vi "systemErrorClusterReplacementCore.vi"(8 "error in (no error)":errorcluster, 11 "Folder Path":path) -> (0 "error out":errorcluster)   [LabVIEW 2017, in "vi_tools.lvlib"]
doc: "From the front panel or block diagram window of a VI or a VI is selected on the File Dialog, select <b>Tools»System Error Cluster Replacement</b> to replace all Error clusters (in and out) on the VI front panel with System Error cluster.\n\nFrom the a project or lvlib explorer window or a folder is selected on the File Dialog, select <b>Tools»System Error Cluster Replacement</b> to replace all Error clusters (in and out) on all VI front panels with System Error cluster within the project or lvlib or user selected folder on disk."
uses:
  <vilib>/Utility/traverseref.llb/TRef TravTarget.ctl
  vi_tools.lvlib
panel:
  out "progress":string
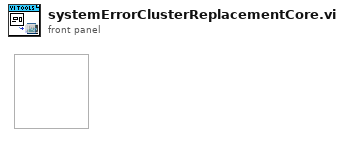
[diagram p1: front panel]
types:
  T1 = enum32{"Invalid", "Standard", "Closed", "Hidden", "Minimized", "Maximized"}
  T2 = typedef "TRef TravTarget.ctl" = enum16{"FP", "BD", "Other"}
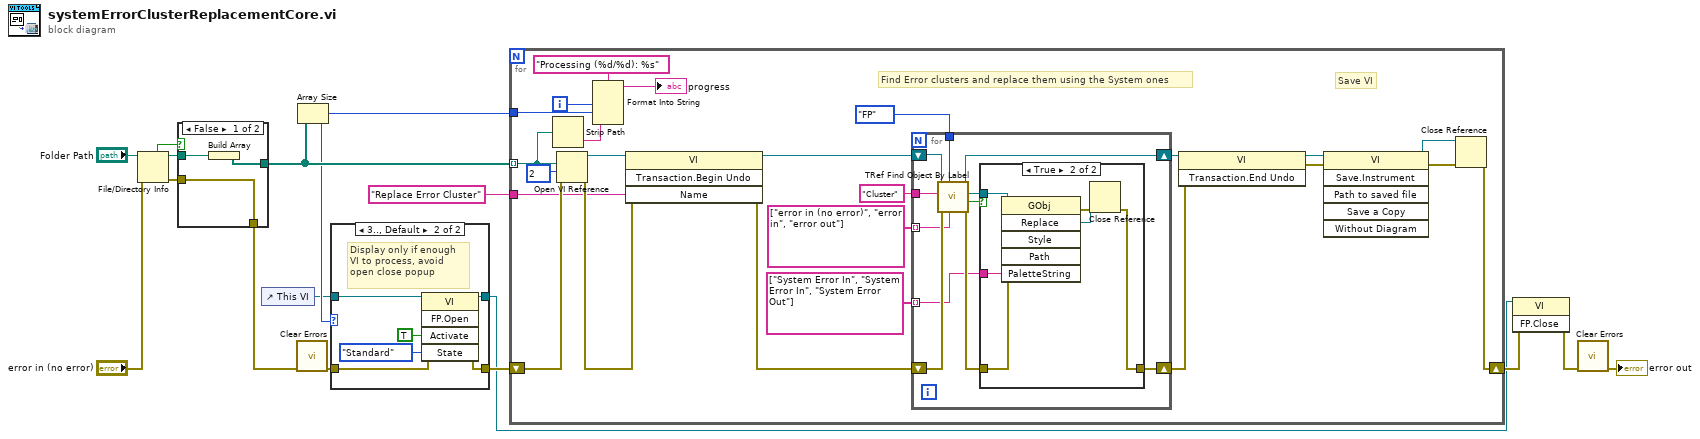
[diagram p0: block diagram]
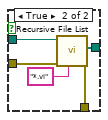
[diagram p2: hidden frame]
diagram:
  n1 = File/Directory Info(path="Folder Path", error in="error in (no error)") -> (path out=w10:path, directory=w8:bool, error out=w9:errorcluster)  [unwired: 4 out]
  n2 = case shown="False" w8 {
    tunnel: [w17 w23] -> w16
    tunnel: [w18 w22] -> w15
    tunnel: w10 -> [w19 w21]
    tunnel: w9 -> [w18 w20]
    frame False {
      n3 = Build Array(w19) -> (w17:path[])
    }
    frame True {
      n4 = call <vilib>:"Recursive File List.vi"("pattern"="*.vi", "error in (no error)"=w20, "Folder Path"=w21) -> ("error out"=w22:errorcluster, "All Files in Dir"=w23:path[])  [unwired: 4 in, 3 out]
    }
  }
  n5 = control-ref of="This VI"() -> (w2:refnum<vi>)
  n6 = call <vilib>:"Clear Errors.vi"("error in (no error)"=w15) -> ("error out"=w3:errorcluster)  [unwired: 5 in, 1 out]
  n7 = Array Size(array=w16) -> (size(s)=w4:i32)
  n8 = case shown="3.., Default" w4 {
    tunnel: w3 -> [w26 w30]
    tunnel: [w26 w29] -> w14
    tunnel: w2 -> [w25 w28]
    tunnel: [w25 w27] -> w5
    frame 0..2 {
    }
    frame 3.., Default {
      # "Display only if enough\nVI to process, avoid \nopen close popup"
      n9 = invoke class="VI" method="FP.Open"(reference=w28, error in=w30, "Activate"=TRUE ("Activate?"), "State"=T1."Standard") -> (reference out=w27:refnum<vi>, error out=w29:errorcluster)  [unwired: 1 in, 3 out]
    }
  }
  n10 = for {
    shift-right: [w49] -> w13
    shift-left: w14 -> [w47]
    tunnel: w16 -> [w45] mode=indexing
    tunnel: w4 -> [w42]
    tunnel: "Replace Error Cluster" ("Name") -> [w36]
    i -> [w44]
    # "Save VI"
    # "Find Error clusters and replace them using the System ones"
    n11 = Strip Path(path=w45) -> (name=w41:string)  [unwired: 1 out]
    n12 = Open VI Reference(vi path=w45, options=2, error in (no error)=w47) -> (vi reference=w48:refnum<vi>, error out=w38:errorcluster)  [unwired: 3 in]
    n13 = Format Into String(format string="Processing (%d/%d): %s", w44, w42, w41) -> (resulting string=→"progress":string)  [unwired: 2 in, 1 out]
    n14 = invoke class="VI" method="Transaction.Begin Undo"(reference=w48, error in=w38, "Name"=w36) -> (reference out=w39:refnum<vi>, error out=w37:errorcluster)  [unwired: 1 in, 2 out]
    n15 = for {
      tunnel: TRef_TravTarget."FP" ("Traverse Target") -> [w66]
      tunnel: "Cluster" ("Class Name") -> [w65]
      shift-right: [w62] -> w52
      shift-left: w39 -> [w67]
      tunnel: string[] ["error in (no error)", "error in", "error out"] -> [w58] mode=indexing
      tunnel: string[] ["System Error In", "System Error In", "System Error Out"] -> [w57] mode=indexing
      shift-right: [w61] -> w51
      shift-left: w37 -> [w59]
      n16 = call <vilib>:"TRef Find Object By Label.vi"("Label"=w58, "Traverse Target"=w66, "error in (no error)"=w59, "Class Name"=w65, "VI Ref"=w67) -> ("error out"=w63:errorcluster, "Found?"=w60:bool, "Found Obj Ref"=w64:refnum<vi>, "dup VI Ref"=w62:refnum<vi>)  [unwired: 3 in]
      n17 = case shown="True" w60 {
        tunnel: w64 -> [_ w74]
        tunnel: w63 -> [w68 w73]
        tunnel: w57 -> [_ w72]
        tunnel: [w68 w70] -> w61
        frame False {
        }
        frame True {
          n18 = invoke class="GObj" method="Replace"(reference=w74, error in=w73, "PaletteString"=w72) -> (error out=w71:errorcluster, "Replace"=w69:refnum<vi>)  [unwired: 3 in, 4 out]
          n19 = Close Reference(reference=w69, error in (no error)=w71) -> (error out=w70:errorcluster)
        }
      }
    }
    n20 = invoke class="VI" method="Transaction.End Undo"(reference=w52, error in=w51) -> (reference out=w50:refnum<vi>, error out=w33:errorcluster)  [unwired: 1 in, 1 out]
    n21 = invoke class="VI" method="Save.Instrument"(reference=w50, error in=w33) -> (reference out=w35:refnum<vi>, error out=w34:errorcluster)  [unwired: 4 in, 4 out]
    n22 = Close Reference(reference=w35, error in (no error)=w34) -> (error out=w49:errorcluster)
  }
  n23 = invoke class="VI" method="FP.Close"(reference=w5, error in=w13) -> (error out=w6:errorcluster)  [unwired: 1 in, 2 out]
  n24 = call <vilib>:"Clear Errors.vi"("error in (no error)"=w6) -> ("error out"=→"error out":errorcluster)  [unwired: 5 in, 1 out]
